vi "Summary String.vi"(4 "Obstacle Mode":u16(ring)=1 items=["In a large, open space", "In a small, packed place", "Actual disaster recovery"], 5 "Camera Port 2":refnum<k21>="cam0" caption="Session In", 6 "Obstacle??":enum32{"Radio Selection 1", "Radio Selection 2"}(radio), 7 "Camera YN":enum32{"Radio Selection 1", "Radio Selection 2"}(radio), 8 "Arm Type":enum32{"RS1", "RS2"}(radio), 9 "Mode out":enum8{"Protected Manaul", "Automatic", "Manaul"}(ring)=enum."Manaul", 10 "Servo Frequency [Hz]":u32=20000) -> (2 "String":T1="Mode:\n\nArm:\n\nCamera\n\nObstacle Y/N:\nObstacle Mode: ")   [LabVIEW 2015]
uses:
  Controls/Summary String.ctl
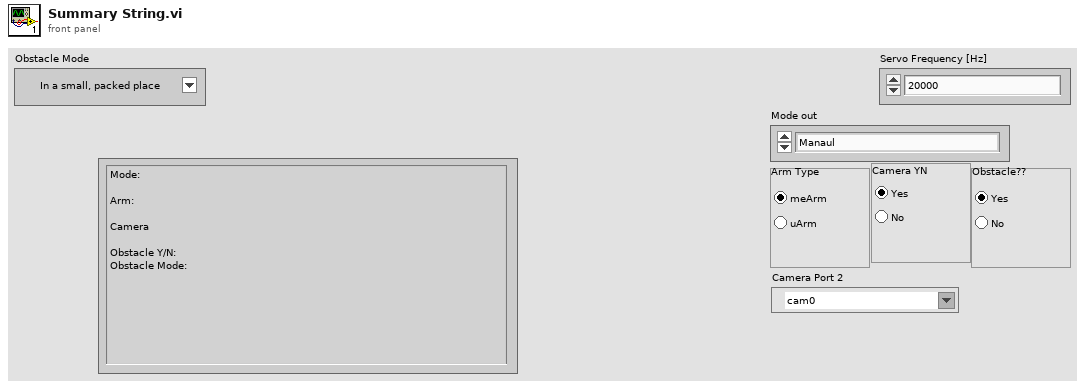
[diagram p1: front panel]
types:
  T1 = typedef "Summary String.ctl" = string
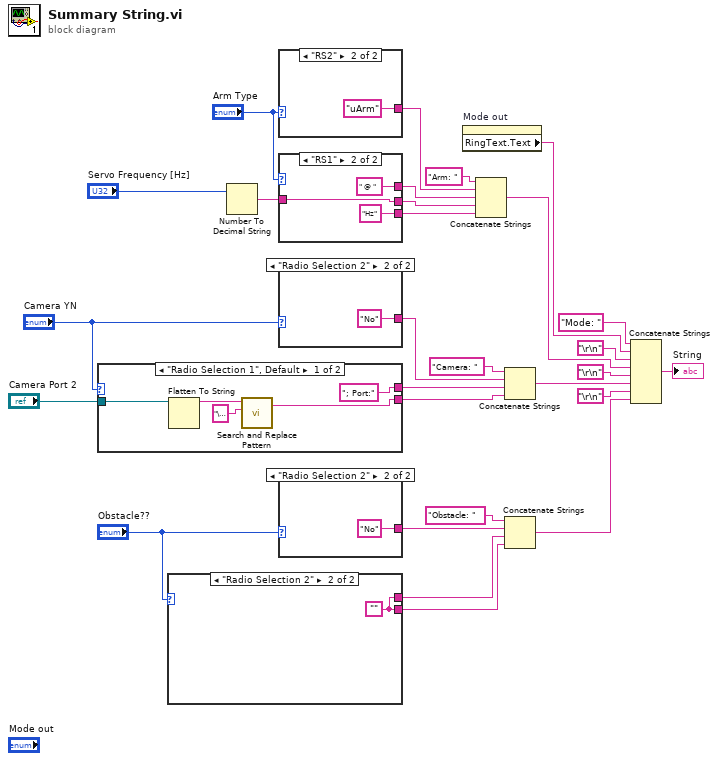
[diagram p0: block diagram]
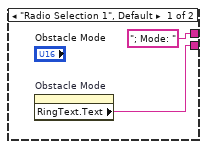
[diagram p2: hidden frame]
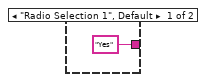
[diagram p3: hidden frame]
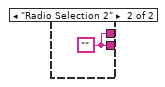
[diagram p4: hidden frame]
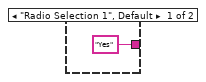
[diagram p5: hidden frame]
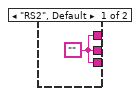
[diagram p6: hidden frame]
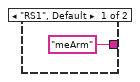
[diagram p7: hidden frame]
diagram:
  n1 = case shown="\"Radio Selection 1\", Default" "Camera YN" {
    tunnel: ["; Port:" w34] -> w7
    tunnel: "Camera Port 2" -> [w32 _]
    tunnel: [w30 w34] -> w5
    frame "Radio Selection 1", Default {
      n2 = Flatten To String(anything=w32) -> (data string=w31:string)  [unwired: 3 in, 2 out]
      n3 = call <vilib>:"Search and Replace Pattern.vi"("string"=w31, "regular expression (\"\")"="\u0004" ("regular expression (\"\")")) -> ("result string"=w30:string)  [unwired: 3 in, 1 out]
    }
    frame "Radio Selection 2" {
      w34 = ""
    }
  }
  n4 = case shown="\"Radio Selection 2\"" "Obstacle??" {
    tunnel: ["; Mode: " w37] -> w2
    tunnel: [w35 w37] -> w1
    frame "Radio Selection 1", Default {
      n5 = property on="Obstacle Mode" class="Ring (strict)"() -> ("RingText.Text"=w35:string)  [unwired: 2 in, 2 out]
    }
    frame "Radio Selection 2" {
      w37 = ""
    }
  }
  n6 = Number To Decimal String(number="Servo Frequency [Hz]") -> (decimal integer string=w11:string)  [unwired: 1 in]
  n7 = case shown="\"RS2\"" "Arm Type" {
    tunnel: ["meArm" "uArm"] -> w14
    frame "RS1", Default {
    }
    frame "RS2" {
    }
  }
  n8 = case shown="\"RS1\"" "Arm Type" {
    tunnel: [w40 " @ "] -> w27
    tunnel: [w40 "Hz"] -> w26
    tunnel: [w40 w41] -> w12
    tunnel: w11 -> [_ w41]
    frame "RS2", Default {
      w40 = ""
    }
    frame "RS1" {
    }
  }
  n9 = case shown="\"Radio Selection 2\"" "Camera YN" {
    tunnel: ["Yes" "No"] -> w9
    frame "Radio Selection 1", Default {
    }
    frame "Radio Selection 2" {
    }
  }
  n10 = case shown="\"Radio Selection 2\"" "Obstacle??" {
    tunnel: ["Yes" "No"] -> w4
    frame "Radio Selection 1", Default {
    }
    frame "Radio Selection 2" {
    }
  }
  n11 = property on="Mode out" class="Enum (strict)"() -> ("RingText.Text"=w15:string)  [unwired: 2 in, 2 out]
  n12 = Concatenate Strings("Arm: ", w14, w27, w12, w26) -> (w21:string)
  n13 = Concatenate Strings("Camera: ", w9, w7, w5) -> (w19:string)
  n14 = Concatenate Strings("Obstacle: ", w4, w2, w1) -> (w17:string)
  n15 = Concatenate Strings("Mode: ", w15, "\r\n", w21, "\r\n", w19, "\r\n", w17) -> (→"String":string)
